vi "Error_Logger.vi"(11 "Error_In":errorcluster) -> (4 "Error_Table":string[][](table) caption="Error Table", 15 "Error_Out":errorcluster)   [LabVIEW 2023]
doc: "This VI Shows the Error data of current and temperature."
uses:
  Controls/Error_Data.ctl
  Controls/Queue_Operation_Select.ctl
  Controls/State_and_Data.ctl
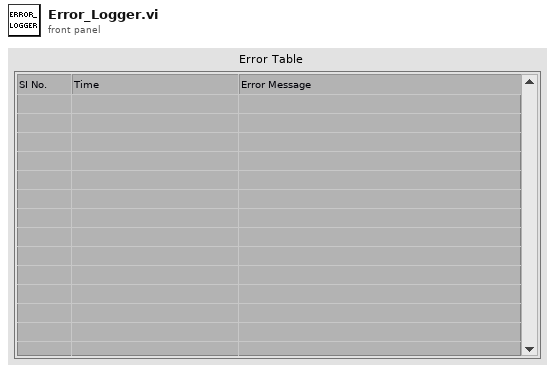
[diagram p1: front panel]
types:
  T1 = typedef "Queue_Operation_Select.ctl" = enum16{"Obtain_Queue", "Enqueue", "Enqueue_N", "Lossy_Enqueue", "Preview", "Queue_Status", "Release_Queue", "Dequeue", "Flush"}
  T2 = enum32{"Invalid", "Standard", "Closed", "Hidden", "Minimized", "Maximized"}
  T3 = typedef "Error_Data.ctl" = cluster{"Error_Table_Data":string[][], "SI_No":i32, "Log_Rate":u32}
  T4 = typedef "State_and_Data.ctl" = cluster{"State":string, "Data":variant}
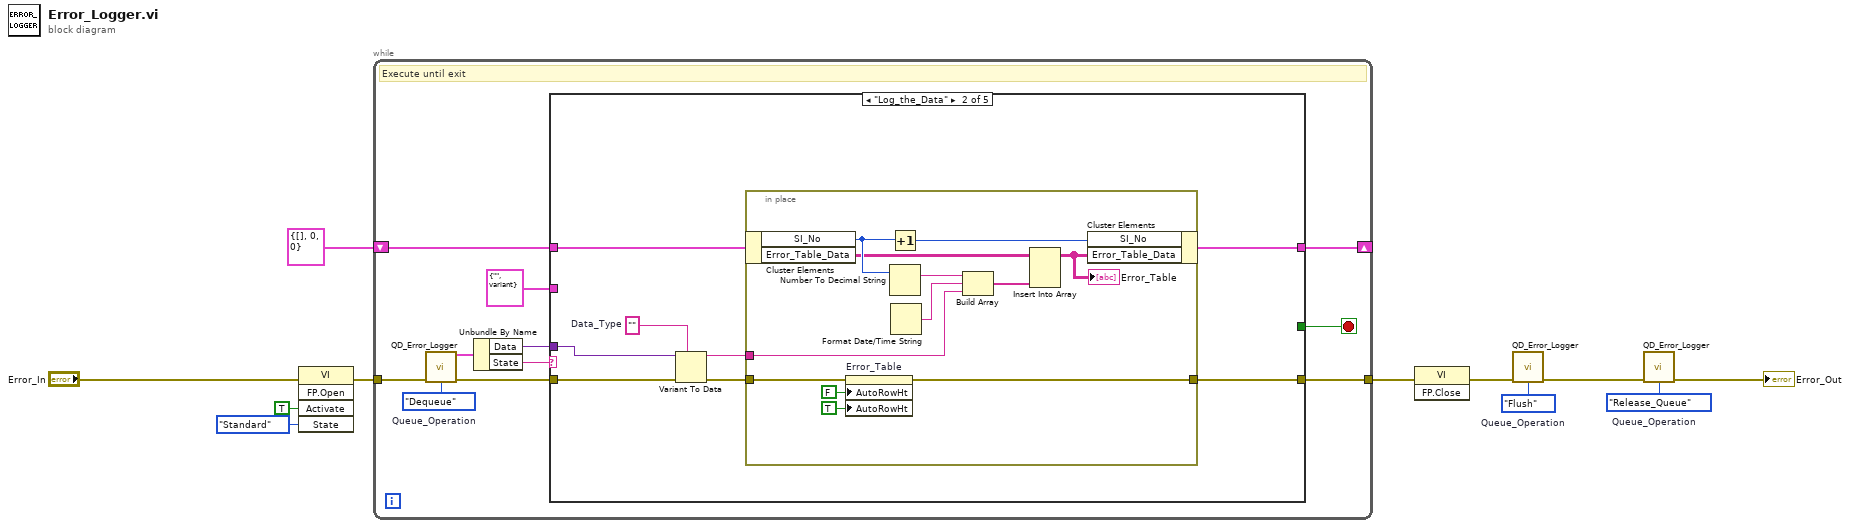
[diagram p0: block diagram]
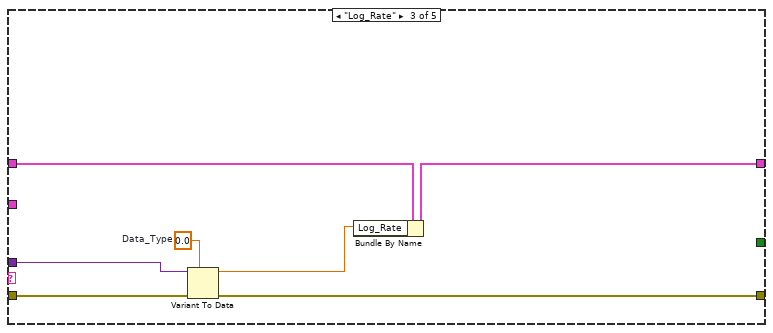
[diagram p3: hidden frame]
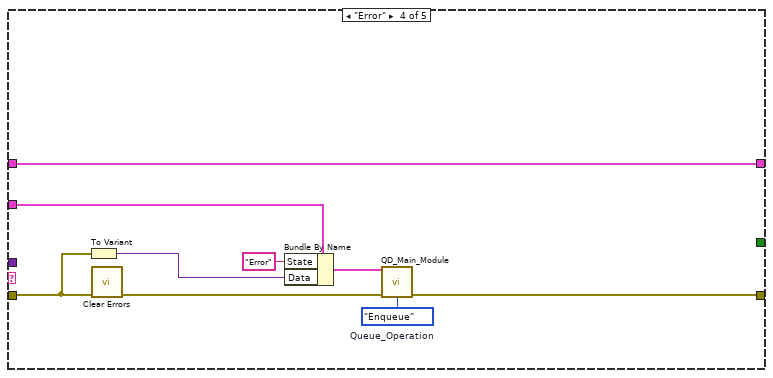
[diagram p4: hidden frame]
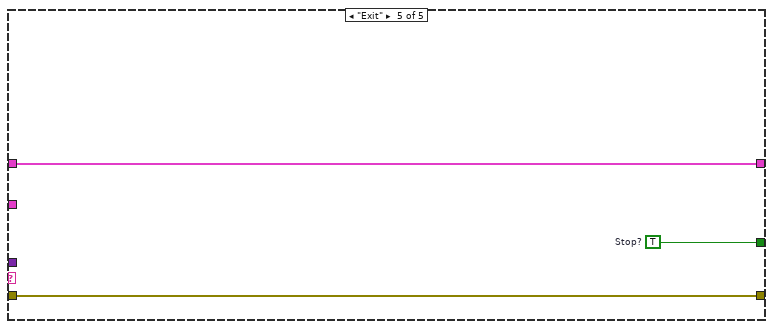
[diagram p5: hidden frame]
diagram:
  w2 = Queue_Operation_Select."Release_Queue"  # Queue_Operation
  w6 = Queue_Operation_Select."Flush"  # Queue_Operation
  n1 = invoke class="VI" method="FP.Open"(error in="Error_In", "Activate"=TRUE ("Activate?"), "State"=T2."Standard") -> (error out=w10:errorcluster)  [unwired: 2 in, 4 out]
  n2 = while {
    shift-right: [w21] -> _
    shift-left: T3 {"Error_Table_Data"=[], "SI_No"=0, "Log_Rate"=0} -> [w22]
    tunnel: w10 -> [w17]
    tunnel: [w20] -> w7
    stop <- w12 stop-if-true
    w15 = Queue_Operation_Select."Dequeue"  # Queue_Operation
    # "Execute until exit"
    n3 = call "QD_Error_Logger.vi"("Error_In"=w17, "Queue_Operation"=w15) -> ("State_and_Data_Out"=w14:T4, "Error_Out"=w16:errorcluster)  [unwired: 12 in]
    n4 = Unbundle By Name(w14) -> ("Data"=w18:variant, "State"=w19:string)
    n5 = case shown="\"Log_the_Data\"" w19 {
      tunnel: w22 -> [w24 w25 w50 w60 w63]
      tunnel: [w24 w32 w49 w60 w63] -> w21
      tunnel: [w23 w31 w48 w53 w62] -> w20
      tunnel: w16 -> [w23 w30 w51 w54 w62]
      tunnel: w18 -> [_ w28 w47 _ _]
      tunnel: T4 {"State"="", "Data"=variant} ("State_and_Data_In") -> [_ _ _ w52 _]
      tunnel: [_ _ _ _ w61] -> w12
      frame Default {
      }
      frame "Log_the_Data" {
        w27 = ""  # Data_Type
        n6 = Variant To Data(error in=w30, type=w27, Variant=w28) -> (data=w26:string, error out=w29:errorcluster)
        n7 = in-place {
          in-place-border: [w33] -> w31
          in-place-border: w29 -> [w34]
          in-place-border: w26 -> [w35]
          n8 = in-place-cluster #1(w25) -> ("SI_No"=w42:i32, "Error_Table_Data"=w41:string[][])
          n9 = property on="Error_Table" class="Tbl (strict)"(error in=w34, "AutoRowHt"=FALSE ("Autosizing Row Height"), "AutoRowHt"=TRUE ("Autosizing Row Height")) -> (error out=w33:errorcluster)  [unwired: 1 in, 1 out]
          n10 = Increment(x=w42) -> (x+1=w40:i32)
          n11 = Number To Decimal String(number=w42) -> (decimal integer string=w44:string)  [unwired: 1 in]
          n12 = Format Date/Time String() -> (date/time string=w43:string)  [unwired: 3 in]
          n13 = Build Array(w44, w43, w35) -> (w36:string[])
          n14 = Insert Into Array(array=w41, new element=w36) -> (w37:string[][])  [unwired: 2 in]
          "Error_Table" <- w37
          n15 = in-place-cluster #1("SI_No"=w40, "Error_Table_Data"=w37) -> (w32:T3)
        }
      }
      frame "Log_Rate" {
        w46 = 0.0  # Data_Type
        n16 = Variant To Data(error in=w51, type=w46, Variant=w47) -> (data=w45:dbl, error out=w48:errorcluster)
        n17 = Bundle By Name(cluster=w50, "Log_Rate"=w45) -> (w49:T3)
      }
      frame "Error" {
        w59 = Queue_Operation_Select."Enqueue"  # Queue_Operation
        n18 = To Variant(anything=w54) -> (Variant=w56:variant)
        n19 = call <vilib>:"Clear Errors.vi"("error in (no error)"=w54) -> ("error out"=w55:errorcluster)  [unwired: 5 in, 1 out]
        n20 = Bundle By Name(cluster=w52, "State"="Error", "Data"=w56) -> (w58:T4)
        n21 = call "QD_Main_Module.vi"("Data_In"=w58, "Error_In"=w55, "Queue_Operation"=w59) -> ("Error_Out"=w53:errorcluster)  [unwired: 8 in, 4 out]
      }
      frame "Exit" {
        w61 = TRUE  # Stop?
      }
    }
  }
  n22 = invoke class="VI" method="FP.Close"(error in=w7) -> (error out=w5:errorcluster)  [unwired: 2 in, 2 out]
  n23 = call "QD_Error_Logger.vi"("Error_In"=w5, "Queue_Operation"=w6) -> ("Error_Out"=w4:errorcluster)  [unwired: 12 in, 1 out]
  n24 = call "QD_Error_Logger.vi"("Error_In"=w4, "Queue_Operation"=w2) -> ("Error_Out"=→"Error_Out":errorcluster)  [unwired: 12 in, 1 out]
